vi "Obtain Group.vi"(8 "error in (no error)":errorcluster, 10 "Group":string, 11 "PrefsDB in (Singleton)":refnum<class "PrefsDB.lvclass">) -> (0 "error out":errorcluster, 2 "Pref Group":refnum<class "Pref Group.lvclass">, 3 "PrefsDB out":refnum<class "PrefsDB.lvclass">)   [LabVIEW 2020, in "User Prefs.lvlib" / "PrefsDB.lvclass"]
uses:
  PrefsDB.lvclass
  Pref Group/Pref Group.lvclass
  Obtain Group Data.ctl
  lv-promises/Promises/Promise/Promise.lvclass
  PrefsDB.lvclass/PrefsDB.ctl
  lv-promises/Promises/Promise/Promise.lvclass/Promise.ctl
  lv-promises/Promises/Future/Future.lvclass/Future.ctl
  Is Valid.vi
  Obtain UserPrefs.vi
  lv-promises/Promises/Future/Future.lvclass
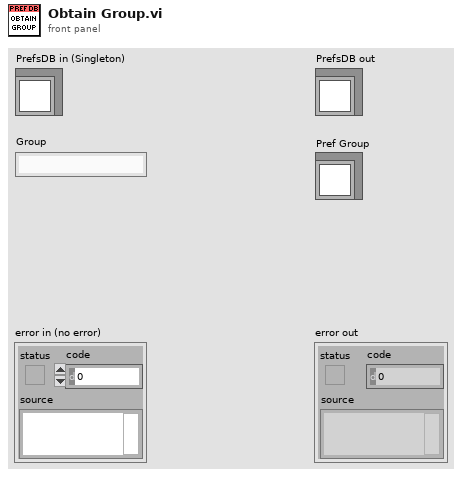
[diagram p1: front panel]
types:
  T1 = typedef "User Prefs.lvlib/PrefsDB.lvclass/Obtain Group Data.ctl" = cluster{"Group Name":string, "Promise":refnum<class "Promise.lvclass">}
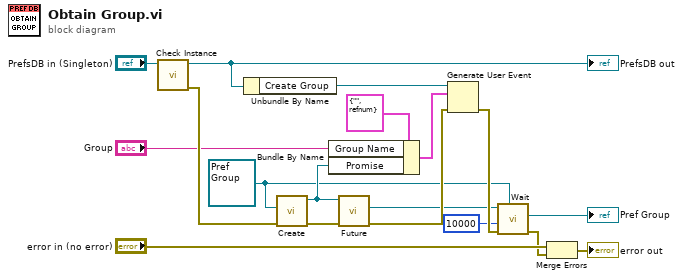
[diagram p0: block diagram]
diagram:
  w1 = refnum<class "Pref Group.lvclass"> refnum ("User Prefs.lvlib:Pref Group.lvclass")
  n1 = call "Check Instance.vi"("PrefsDB in"="PrefsDB in (Singleton)") -> ("error out"=w17:errorcluster, "PrefsDB out"=w2:refnum<class "PrefsDB.lvclass">)  [unwired: 9 in]
  "PrefsDB out" <- w2
  n2 = Unbundle By Name(w2) -> ("Create Group"=w9:refnum<user-event>)
  n3 = call "Create.vi"("error in (no error)"=w17, "Result Type (None)"=w1) -> ("error out"=w15:errorcluster, "Promise"=w7:refnum<class "Promise.lvclass">)  [unwired: 8 in]
  n4 = Bundle By Name(cluster=T1 {"Group Name"="", "Promise"=refnum} ("Obtain Group Data"), "Group Name"="Group", "Promise"=w7) -> (w8:T1)
  n5 = call "Future.vi"("Promise in"=w7) -> ("Future"=w6:refnum<class "Future.lvclass">)  [unwired: 9 in, 1 out]
  n6 = Generate User Event(user event=w9, event data cluster=w8, error in=w15) -> (error out=w16:errorcluster)  [unwired: 1 in, 1 out]
  n7 = call "Wait.vi"("Result Type (None)"=w1, "error in (no error)"=w16, "Timeout mS (-1)"=10000, "Future in"=w6) -> ("error out"=w4:errorcluster, "Result"=→"Pref Group":refnum<class "Pref Group.lvclass">)  [unwired: 6 in]
  n8 = Merge Errors("error in (no error)", w4) -> (→"error out":errorcluster)
